vi "1 filtre ds tab historique.vi"(3 "Filtre":T1(ring), 4 "valeur recherchée":string) -> (0 "Tab historique filtré par ordre croissant carton":string[][](array[string]), 1 "Tab historique filtré":string[][](array[string]))   [LabVIEW 2020]
doc: "Renvoie le tableau historique des pièces qui contiennent la valeur du filtre recherchée dans l'historique des valves emballées.\nOn peut filtrer sur le n° du produit, la date d'emballage, l'opérateur, le n° de cmde ou le n° du carton.\n\nComposition des colonnes :\n colonne 0 : n° des pièces (code bar 18 chiffres)\n colonne 1 : date\n colonne 2 : visa emballage (n°)\n colonne 3 : n° commande (complet)\n colonne 4 : n° carton\n colonne 5 : qtté totale de la cmde"
uses:
  Modules/FS/60_FS_Controles/60_FS_SetGet.ctl
panel:
  out "tab historique":string[][](array[string])
  # "0"
  # "1"
  # "2"
  # "3"
  # "4"
  # "5"
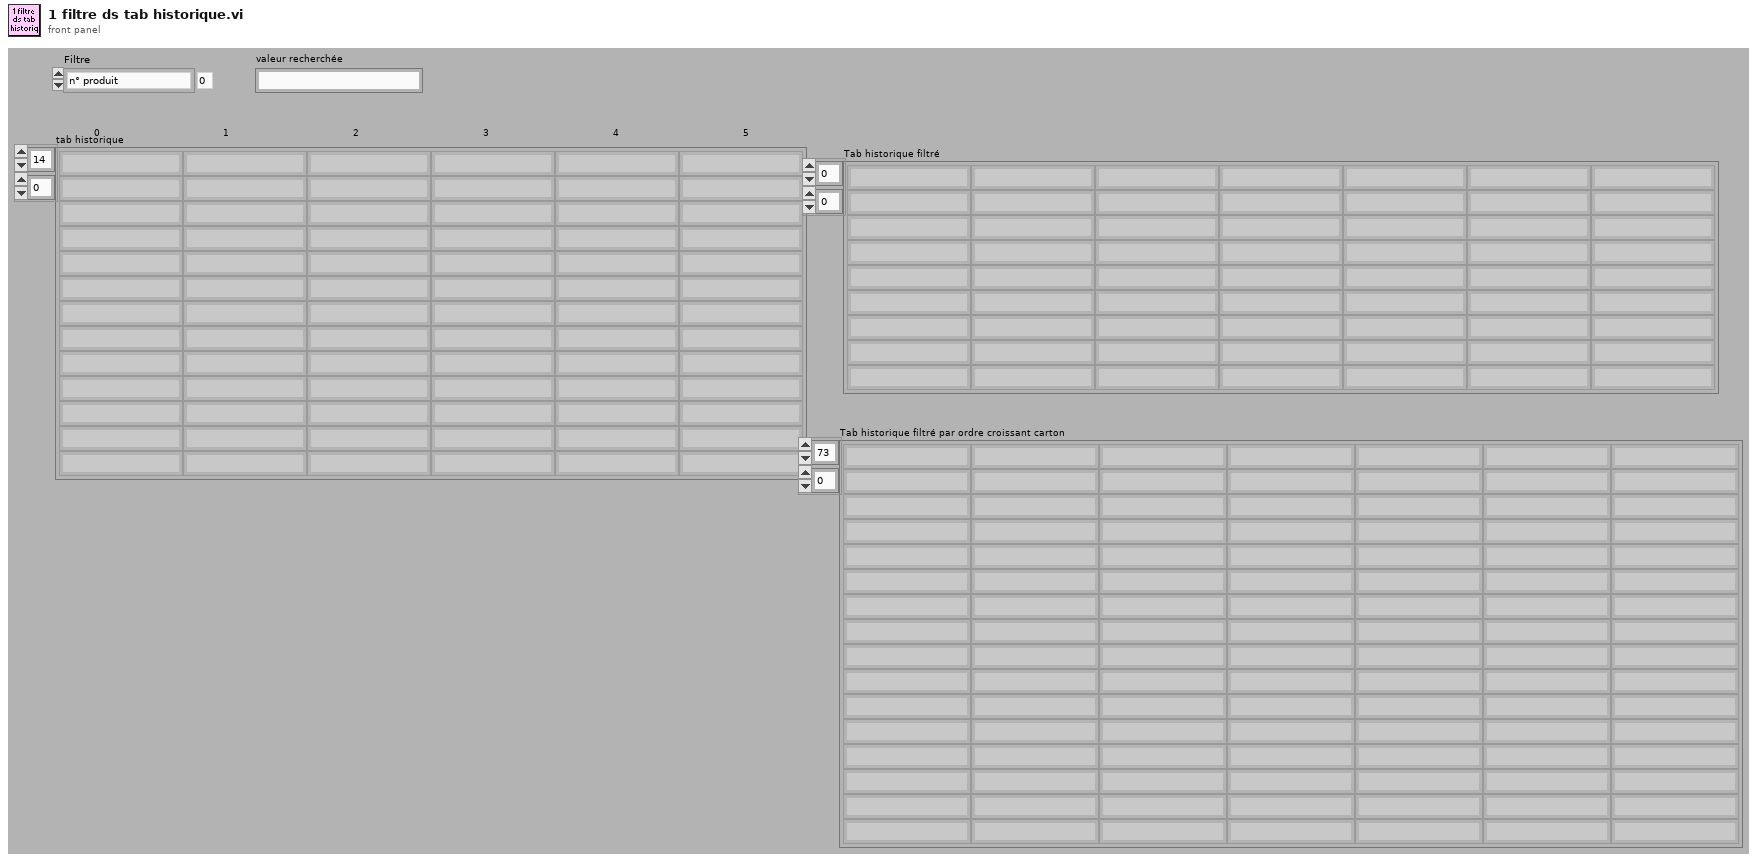
[diagram p1: front panel]
types:
  T1 = enum16{"n° produit", "date", "opérateur", "n° cmde", "n° carton", "qtté cmdée ou retour client"}
  T2 = typedef "60_FS_SetGet.ctl" = enum16{"set", "get"}
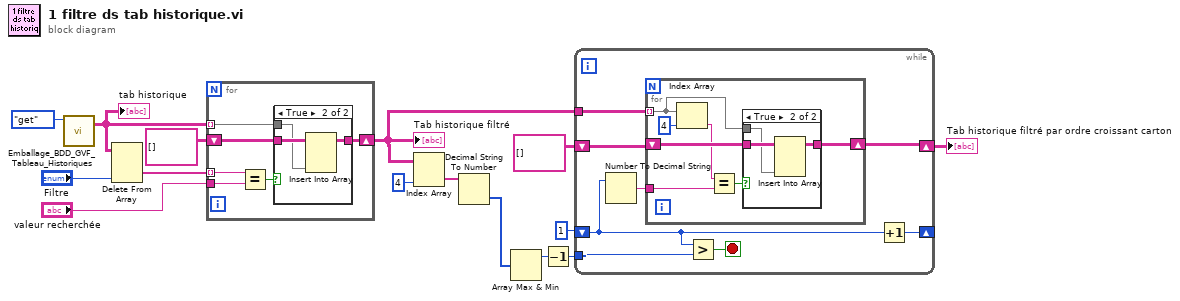
[diagram p0: block diagram]
diagram:
  n1 = call "Emballage_BDD_GVF_Tableau_Historiques.vi"("SetGet"=60_FS_SetGet."get") -> ("Tableau historique OUT"=w5:string[][])  [unwired: 9 in, 1 out]
  "tab historique" <- w5
  n2 = Delete From Array(array=w5, index (col)="Filtre") -> (deleted portion=w15:string[])  [unwired: 2 in, 1 out]
  n3 = for {
    tunnel: w15 -> [w20] mode=indexing
    tunnel: "valeur recherchée" -> [w21]
    shift-right: [w17] -> w9
    shift-left: string[][] [] -> [w16]
    tunnel: w5 -> [w18] mode=indexing
    n4 = Equal?(x=w20, y=w21) -> (x = y?=w19:bool)
    n5 = case shown="True" w19 {
      tunnel: w18 -> [_ w23]
      tunnel: [w22 w25] -> w17
      tunnel: w16 -> [w22 w24]
      frame False {
      }
      frame True {
        n6 = Insert Into Array(array=w24, new element=w23) -> (w25:string[][])  [unwired: 2 in]
      }
    }
  }
  "Tab historique filtré" <- w9
  n7 = Index Array(array=w9, index (col)=4 ("indice désactivé (col)")) -> (element=w3:string[])  [unwired: 1 in]
  n8 = Decimal String To Number(string=w3) -> (number=w2:i32[])  [unwired: 2 in, 1 out]
  n9 = Array Max & Min(array=w2) -> (max value=w1:i32)  [unwired: 3 out]
  n10 = Decrement(x=w1) -> (x-1=w6:i32)
  n11 = while {
    tunnel: w9 -> [w33]
    shift-right: [w32] -> _
    shift-left: 1 -> [w30]
    shift-right: [w28] -> w8
    shift-left: string[][] [] -> [w29]
    tunnel: w6 -> [w26]
    stop <- w31 stop-if-true
    n12 = Number To Decimal String(number=w30) -> (decimal integer string=w27:string)  [unwired: 1 in]
    n13 = for {
      tunnel: w33 -> [w37] mode=indexing
      shift-right: [w40] -> w28
      shift-left: w29 -> [w39]
      tunnel: w27 -> [w35]
      n14 = Index Array(array=w37, index=4 ("indice désactivé (col)")) -> (element=w34:string)
      n15 = Equal?(x=w34, y=w35) -> (x = y?=w36:bool)
      n16 = case shown="True" w36 {
        tunnel: w37 -> [_ w42]
        tunnel: [w41 w44] -> w40
        tunnel: w39 -> [w41 w43]
        frame False {
        }
        frame True {
          n17 = Insert Into Array(array=w43, new element=w42) -> (w44:string[][])  [unwired: 2 in]
        }
      }
    }
    n18 = Greater?(x=w30, y=w26) -> (0:w31:bool)
    n19 = Increment(x=w30) -> (x+1=w32:i32)
  }
  "Tab historique filtré par ordre croissant carton" <- w8
